vi "Write Data.vi"(8 "error in (no error)":errorcluster, 10 "Base Data Lib:Data":refnum<class "Data.lvclass">, 11 "Test Device in":refnum<class "Test Device.lvclass">) -> (0 "error out":errorcluster, 3 "Test Device out":refnum<class "Test Device.lvclass">)   [LabVIEW 2014, in "Test Device.lvclass"]
uses:
  Test Device.lvclass
  reusable/Data/Data.lvclass
  Test Device.lvclass/Test Device.ctl
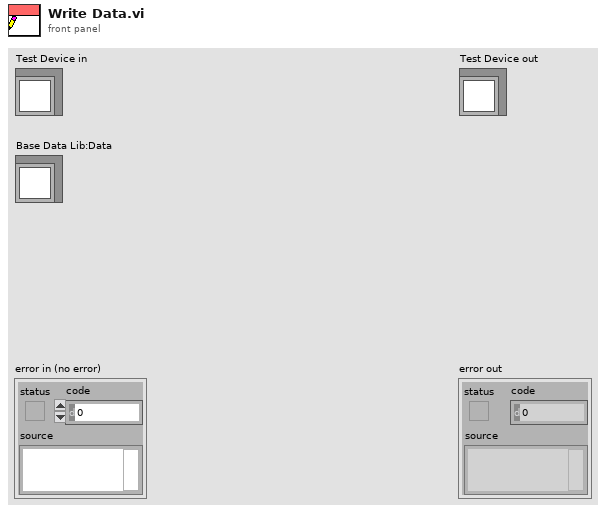
[diagram p1: front panel]
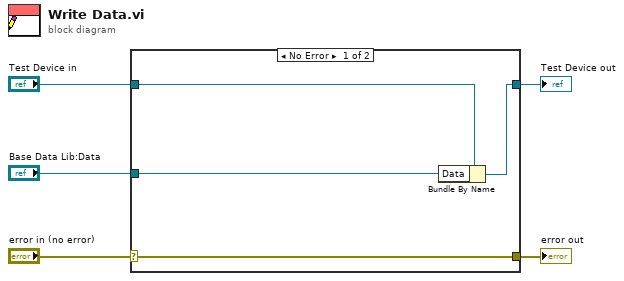
[diagram p0: block diagram]
diagram:
  n1 = case shown="No Error" "error in (no error)" {
    selector: "error in (no error)" -> [w9 w10]
    tunnel: [w9 w10] -> w4
    tunnel: [w7 w11] -> w2
    tunnel: "Test Device in" -> [w8 w11]
    tunnel: "Base Data Lib:Data" -> [w6 _]
    frame No Error {
      n2 = Bundle By Name(cluster=w8, "Data"=w6) -> (w7:refnum<class "Test Device.lvclass">)
    }
    frame Error {
    }
  }
  "error out" <- w4
  "Test Device out" <- w2
